vi "nism.digitalFilter.boolArray(modified).vi"(6 "filter value (us)":u16=2000, 11 "input signal":bool[](array[boolean])=[FALSE, FALSE, FALSE, FALSE, FALSE, FALSE, FALSE, FALSE]) -> (3 "output signal":bool[](array[boolean]))   [LabVIEW 2014]
doc: "Applies the user specified digital filter to the input signal or signals. Filter settings are specified using either the Axis Configuration dialog box or using the appropriate Axis property."
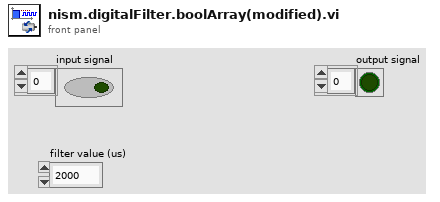
[diagram p1: front panel]
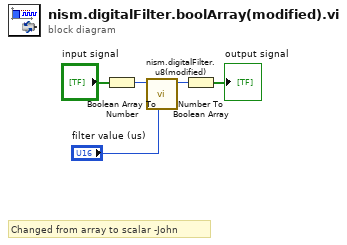
[diagram p0: block diagram]
diagram:
  # "Changed from array to scalar -John"
  n1 = Boolean Array To Number(Boolean array="input signal") -> (number=w3:u8)
  n2 = call "nism.digitalFilter.u8(modified).vi"("filter value (us)"="filter value (us)", "input signal"=w3) -> ("output signal"=w2:u8)  [unwired: 9 in]
  n3 = Number To Boolean Array(number=w2) -> (Boolean array=→"output signal":bool[])
